vi "Merge QoS.vi"(9 "Subscription QoS":T1, 10 "Message QoS":T1) -> (2 "Highest QoS":T1)   [LabVIEW 2013, in "MQTT Server.lvlib" / "Subscription.lvclass"]
uses:
  Subscription.lvclass
  <vilib>/LabVIEW Open Source Project/MQTT Control Packets/Control Packets/ControlPacket/QualityOfService -- enum.ctl
  <vilib>/LabVIEW Open Source Project/MQTT Control Packets/Control Packets/ControlPacket/ControlPacket.lvclass
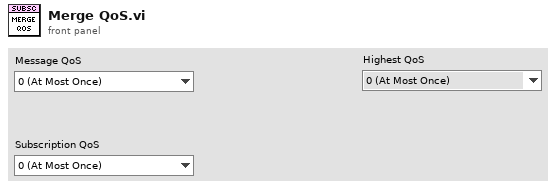
[diagram p1: front panel]
types:
  T1 = typedef "MQTT_Control_Packets.lvlib/ControlPacket.lvclass/QualityOfService -- enum.ctl" = enum16{"0 (At Most Once)", "1 (At Least Once)", "2 (Exactly Once)"}
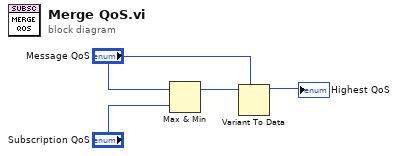
[diagram p0: block diagram]
diagram:
  n1 = Max & Min(x="Message QoS", y="Subscription QoS") -> (max(x,y)=w3:u16)  [unwired: 1 out]
  n2 = Variant To Data(type="Message QoS", Variant=w3) -> (data=→"Highest QoS":T1)  [unwired: 1 in, 1 out]
